vi "Poll.vi"(8 "error in (no error)":errorcluster, 11 "Node Ptr":T2 format="%.0x") -> (0 "error out":errorcluster)   [LabVIEW 2019, in "Diagnostics Addon System Explorer.lvlib"]
uses:
  Diagnostics Addon System Explorer.lvlib
  <vilib>/NI VeriStand/Custom Device API/Custom Device Item Ref.ctl
  Shared/Types/DPID.Rate.ctl
  Types/FG.Action.ctl
  Shared/SubVIs/Constants.vi
  <vilib>/NI VeriStand/Custom Device API/Custom Device API.lvlib
  Shared/Diagnostics Addon Shared.lvlib
panel:
  in  "Speed":T1
  in  "SHDocVw.IWebBrowser":refnum<k7>(container)
  in  "Collection":i32(listbox) caption="Items"
  in  "Description":string
  in  "Name":string
  in  "Header":cluster{"Section Name":string}={"Section Name"="Custom Device Item Settings"}
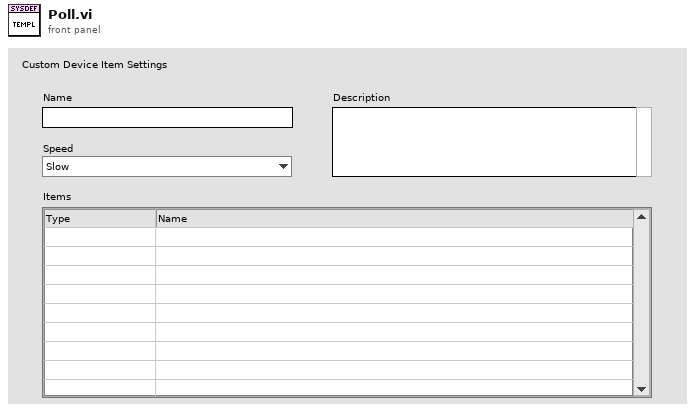
[diagram p1: front panel]
types:
  T1 = typedef "Diagnostics Addon Shared.lvlib/DPID.Rate.ctl" = enum16{"Slow", "Medium", "Fast"}
  T2 = typedef "Custom Device API.lvlib/Custom Device Item Ref.ctl" = u64
  T3 = typedef "Diagnostics Addon System Explorer.lvlib/FG.Action.ctl" = enum16{"Get", "Set"}
  T4 = typedef "Custom Device API.lvlib/Custom Device Item Info.ctl" = cluster{"Name":string, "Is Channel":bool, "GUID":string, "Is Waveform":bool}
  T5 = typedef "Diagnostics Addon System Explorer.lvlib/Poll.Settings.ctl" = cluster{"Input Channels":T6[], "Speed":T1}
  T6 = typedef "Diagnostics Addon System Explorer.lvlib/Poll.LinkedNode.ctl" = cluster{"Node ID":u64}
  T7 = typedef "Custom Device API.lvlib/Custom Device Commands.ctl" = enum16{"Default", "Item renamed", "Shutdown", "Dynamic button pressed"}
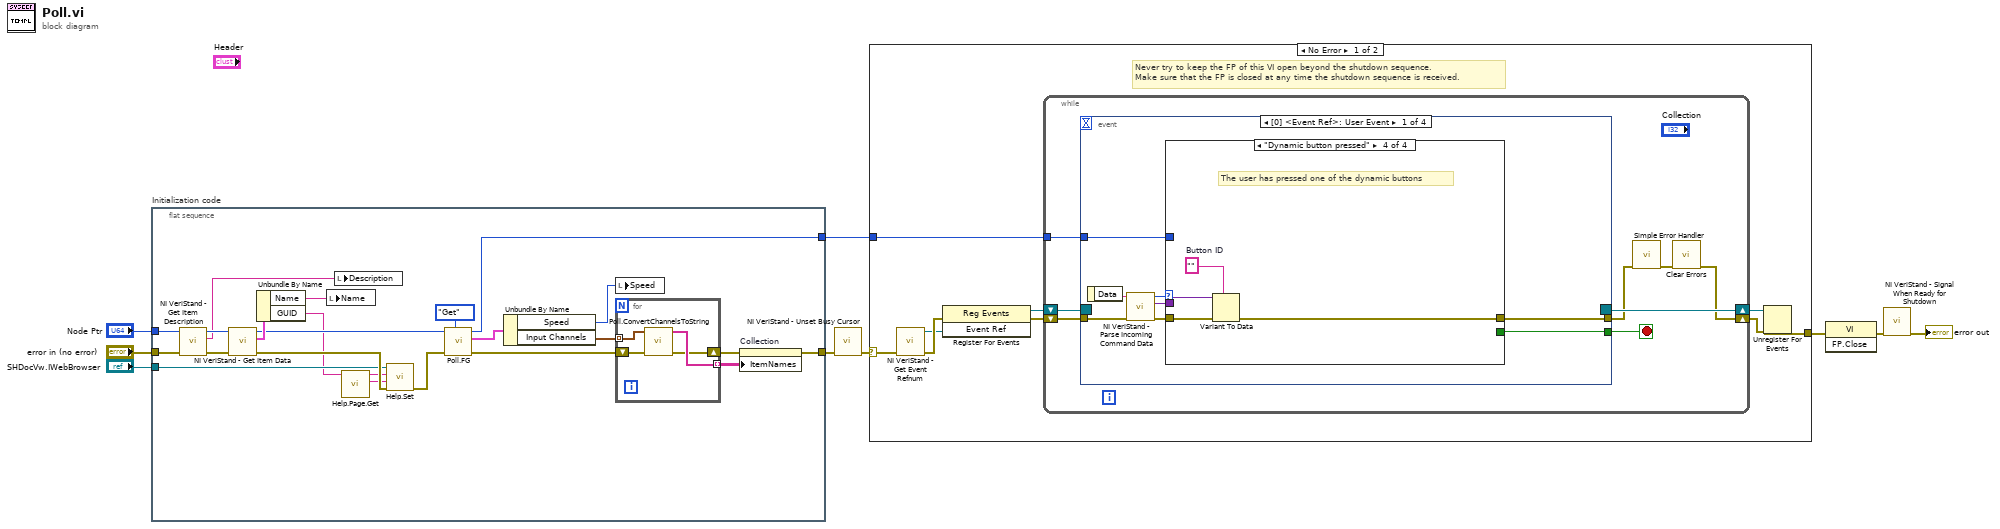
[diagram p0: block diagram]
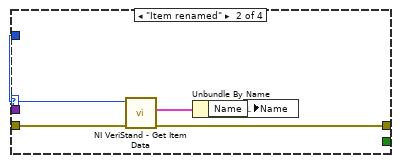
[diagram p3: hidden frame]
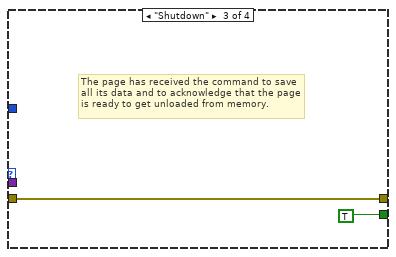
[diagram p4: hidden frame]
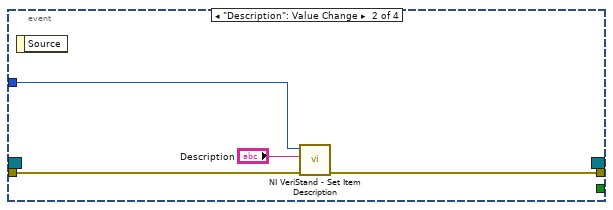
[diagram p5: hidden frame]
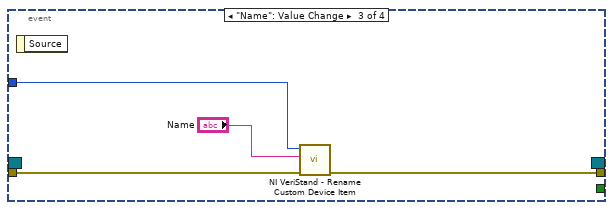
[diagram p6: hidden frame]
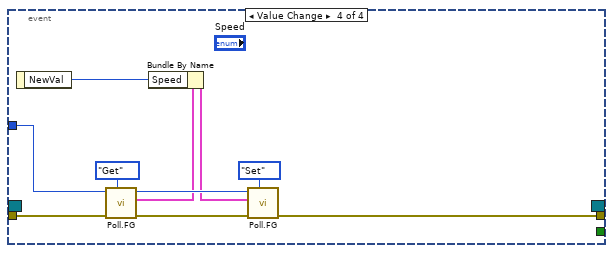
[diagram p7: hidden frame]
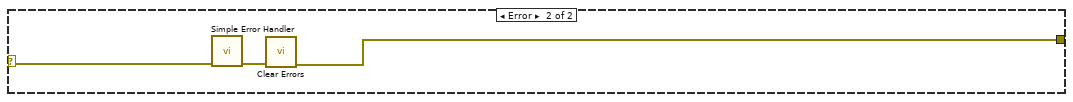
[diagram p8: hidden frame]
diagram:
  n1 = flat-sequence "Initialization code" {
    tunnel: "error in (no error)" -> [w22]
    tunnel: [w26] -> w6
    tunnel: [w17] -> w3
    tunnel: "Node Ptr" -> [w28]
    tunnel: "SHDocVw.IWebBrowser" -> [w23]
    frame #0 {
      n2 = call <vilib>:"NI VeriStand - Get Item Description.vi"("error in (no error)"=w22, "Item Ref in"=w28) -> ("error out"=w30:errorcluster, "Description"=w31:string, "Item Ref out"=w32:T2)  [unwired: 7 out]
      n3 = call <vilib>:"NI VeriStand - Get Item Data.vi"("error in (no error)"=w30, "Item Ref in"=w32) -> ("error out"=w24:errorcluster, "Item Info"=w29:T4, "Item Ref out"=w18:T2)  [unwired: 7 out]
      n4 = Unbundle By Name(w29) -> ("Name"=w14:string, "GUID"=w10:string)
      n5 = local write "Name"(w14) -> ()
      n6 = local write "Description"(w31) -> ()
      n7 = call "Help.Page.Get.vi"("GUID"=w10) -> ("HTML File"=w11:string, "Main CHM File"=w12:string)  [unwired: 9 in]
      n8 = call "Help.Set.vi"("error in (no error)"=w24, "HTML File"=w11, "Main CHM File"=w12, "SHDocVw.IWebBrowser2"=w23) -> ("error out"=w20:errorcluster)  [unwired: 7 in]
      n9 = call "Poll.FG.vi"("Action"=FG.Action."Get", "error in"=w20, "Parent Ref"=w18) -> ("error out"=w19:errorcluster, "Selected Channels out"=w15:T5, "Parent Ref Out"=w17:T2)  [unwired: 6 in]
      n10 = Unbundle By Name(w15) -> ("Speed"=w13:T1, "Input Channels"=w16:T6[])
      n11 = local write "Speed"(w13) -> ()
      n12 = for {
        shift-right: [w33] -> w27
        shift-left: w19 -> [w36]
        tunnel: w16 -> [w35] mode=indexing
        tunnel: [w34] -> w25 mode=indexing
        n13 = call "Poll.ConvertChannelsToString.vi"("error in (no error)"=w36, "MonitoredChannelSettings"=w35) -> ("error out"=w33:errorcluster, "Array"=w34:string[])  [unwired: 8 in]
      }
      n14 = property on="Collection" class="MCListbox (strict)"(error in=w27, "ItemNames"=w25) -> (error out=w26:errorcluster)  [unwired: 1 in, 1 out]
    }
  }
  n15 = call <vilib>:"NI VeriStand - Unset Busy Cursor.vi"("error in (no error)"=w6) -> ("error out"=w5:errorcluster)  [unwired: 10 out]
  n16 = case shown="No Error" w5 {
    selector: w5 -> [w37 w94]
    tunnel: [w42 w92] -> w9
    tunnel: w3 -> [w38 _]
    frame No Error {
      # "Never try to keep the FP of this VI open beyond the shutdown sequence.\nMake sure that the FP is closed at any time the shutdown sequence is received."
      n17 = call <vilib>:"NI VeriStand - Get Event Refnum.vi"("error in (no error)"=w37) -> ("error out"=w45:errorcluster, "Event Ref"=w41:refnum<user-event>)  [unwired: 9 out]
      n18 = register-events(error in=w45, w41) -> (reference out=w39:refnum<event-registration>, error out=w40:errorcluster)  [unwired: 1 in]
      n19 = while {
        tunnel: w38 -> [w49]
        shift-right: [w46] -> w43
        shift-left: w40 -> [w52]
        shift-right: [w53] -> w44
        shift-left: w39 -> [w51]
        stop <- w50 stop-if-true
        n20 = event shown="[0] <Event Ref>: User Event" {
          selector: w51 -> [_ _ _ _]
          dyn-events: [_ _ _ _] -> w53
          timeout: _ -> [_ _ _ _]
          tunnel: w52 -> [w61 w76 w80 w88]
          tunnel: [w57 _ _ _] -> w50
          tunnel: [w56 w75 w79 w85] -> w48
          tunnel: w49 -> [w55 w77 w81 w87]
          event User Event {
            n21 = event-data() -> ("Data"=w60:string)  [unwired: 1 out]
            n22 = call <vilib>:"NI VeriStand - Parse Incoming Command Data.vi"("error in (no error)"=w61, "Incoming data"=w60) -> ("error out"=w59:errorcluster, "Outgoing data"=w54:variant, "Action"=w58:T7)  [unwired: 7 out]
            n23 = case shown="\"Dynamic button pressed\"" w58 {
              tunnel: w59 -> [w62 w67 w68 w73]
              tunnel: [_ _ TRUE _] -> w57
              tunnel: [w62 w64 w68 w70] -> w56
              tunnel: w55 -> [_ w66 _ _]
              tunnel: w54 -> [_ _ _ w72]
              frame "Default", Default {
              }
              frame "Item renamed" {
                n24 = call <vilib>:"NI VeriStand - Get Item Data.vi"("error in (no error)"=w67, "Item Ref in"=w66) -> ("error out"=w64:errorcluster, "Item Info"=w65:T4)  [unwired: 8 out]
                n25 = Unbundle By Name(w65) -> ("Name"=w63:string)
                n26 = local write "Name"(w63) -> ()
              }
              frame "Shutdown" {
                # "The page has received the command to save all its data and to acknowledge that the page is ready to get unloaded from memory."
              }
              frame "Dynamic button pressed" {
                w71 = ""  # Button ID
                # "The user has pressed one of the dynamic buttons"
                n27 = Variant To Data(error in=w73, type=w71, Variant=w72) -> (error out=w70:errorcluster)  [unwired: 1 out]
              }
            }
          }
          event "Description": Value Change {
            n28 = event-data() -> ()  [unwired: 2 out]
            n29 = call <vilib>:"NI VeriStand - Set Item Description.vi"("error in (no error)"=w76, "Description"="Description", "Item Ref in"=w77) -> ("error out"=w75:errorcluster)  [unwired: 8 out]
          }
          event "Name": Value Change {
            n30 = event-data() -> ()  [unwired: 2 out]
            n31 = call <vilib>:"NI VeriStand - Rename Custom Device Item.vi"("error in (no error)"=w80, "New Name"="Name", "Item Ref in"=w81) -> ("error out"=w79:errorcluster)  [unwired: 6 in, 2 out]
          }
          event Value Change {
            n32 = event-data() -> ("NewVal"=w83:T1)  [unwired: 1 out]
            n33 = call "Poll.FG.vi"("Action"=FG.Action."Get", "error in"=w88, "Parent Ref"=w87) -> ("error out"=w89:errorcluster, "Selected Channels out"=w84:T5, "Parent Ref Out"=w86:T2)  [unwired: 6 in]
            n34 = Bundle By Name(cluster=w84, "Speed"=w83) -> (w82:T5)
            n35 = call "Poll.FG.vi"("Action"=FG.Action."Set", "error in"=w89, "Selected Channels"=w82, "Parent Ref"=w86) -> ("error out"=w85:errorcluster)  [unwired: 5 in, 2 out]
          }
        }
        n36 = call <vilib>:"Simple Error Handler.vi"("error in (no error)"=w48) -> ("error out"=w47:errorcluster)  [unwired: 1 in, 7 out]
        n37 = call <vilib>:"Clear Errors.vi"("error in (no error)"=w47) -> ("error out"=w46:errorcluster)  [unwired: 1 in, 5 out]
      }
      n38 = Unregister For Events(event registration refnum=w44, error in=w43) -> (error out=w42:errorcluster)
    }
    frame Error {
      n39 = call <vilib>:"Simple Error Handler.vi"("error in (no error)"=w94) -> ("error out"=w93:errorcluster)  [unwired: 1 in, 7 out]
      n40 = call <vilib>:"Clear Errors.vi"("error in (no error)"=w93) -> ("error out"=w92:errorcluster)  [unwired: 1 in, 5 out]
    }
  }
  n41 = invoke class="VI" method="FP.Close"(error in=w9) -> (error out=w8:errorcluster)  [unwired: 2 in, 2 out]
  n42 = call <vilib>:"NI VeriStand - Signal When Ready for Shutdown.vi"("error in (no error)"=w8) -> ("error out"=→"error out":errorcluster)  [unwired: 10 out]
